vi "clear Session Data.vi"(0 "Session in":refnum<class "SLSC Session.lvclass">, 11 "error in":errorcluster) -> (4 "Session out":refnum<class "SLSC Session.lvclass">, 15 "error out":errorcluster)   [LabVIEW 2015, in "SLSC Switch.lvlib" / "SLSC Session.lvclass"]
uses:
  SLSC Session.lvclass
  SLSC Session.lvclass/SLSC Session.ctl
  <vilib>/SLSC/Close Session.vi
  <vilib>/SLSC/SLSC.lvlib
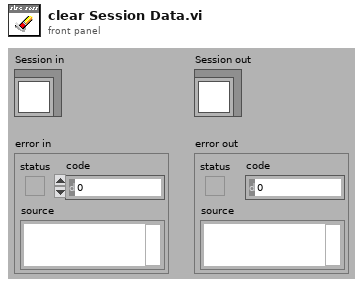
[diagram p1: front panel]
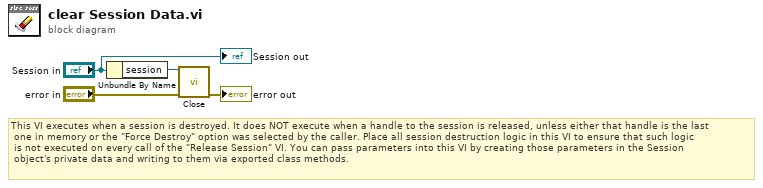
[diagram p0: block diagram]
diagram:
  # "This VI executes when a session is destroyed. It does NOT execute when a handle to the session is released, unless either that handle is the last\n one in memory or the \"Force Destroy\" option was selected by the caller. Place all session destruction logic in this VI to ensure that such logic\n is not executed on every call of the \"Release Session\" VI. You can pass parameters into this VI by creating those parameters in the Session \n object's private data and writing to them via exported class methods."
  n1 = Unbundle By Name("Session in") -> ("session"=w1:refnum<k21>)
  n2 = call-poly <vilib>:"Close.vi"("session in"=w1, "error in (no error)"="error in") -> ("error out"=→"error out":errorcluster)  [unwired: 13 in]
  "Session out" <- "Session in"
